vi "LS370Monitor.vi"() -> ()   [LabVIEW 2015]
uses:
  Instrument_Setup.vi
  Global/Global Variables/global.vi
  Global/Global Variables/Data_Display_global.vi
panel:
  out "Tsweeps Running":bool
  in  "Stopp":bool
  out "MC Heater Output":dbl
  # "Manuelle Steuerung"
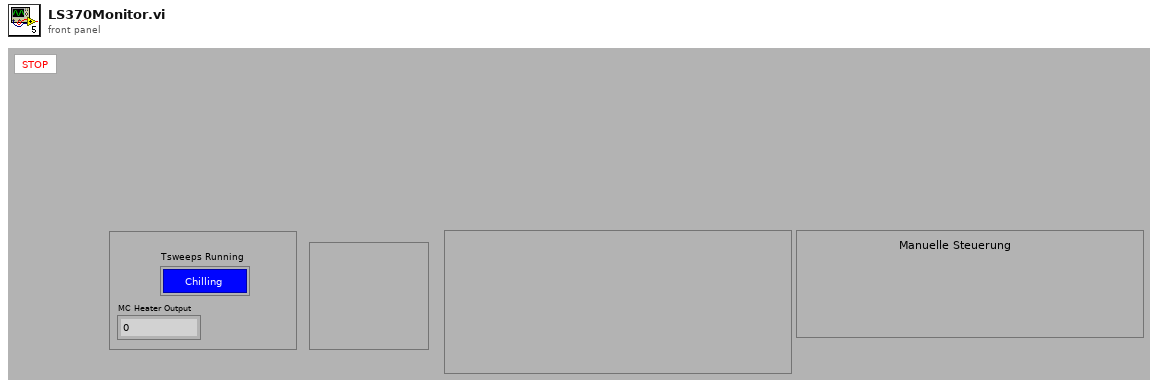
[diagram p1: front panel]
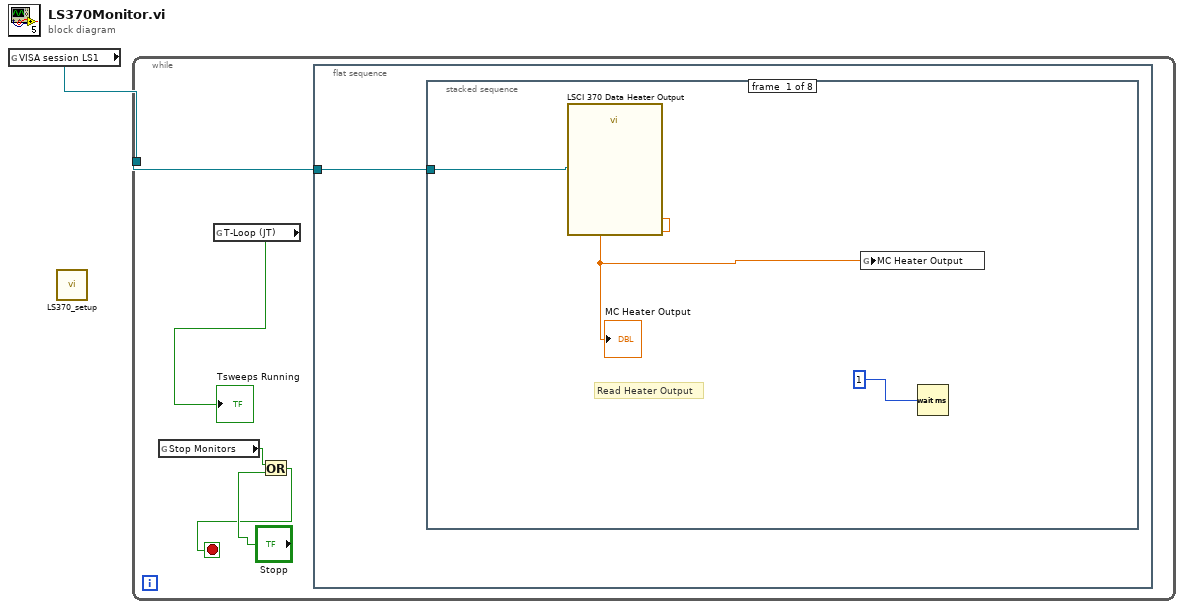
[diagram p0: block diagram]
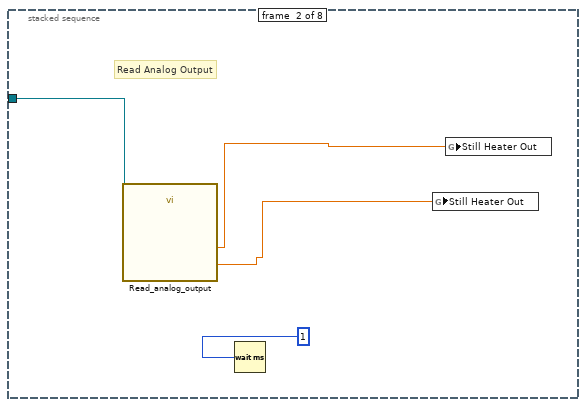
[diagram p2: hidden frame]
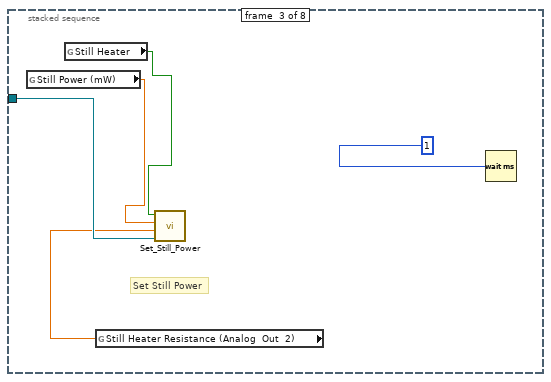
[diagram p3: hidden frame]
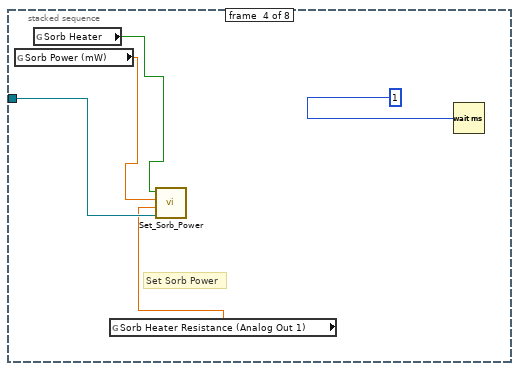
[diagram p4: hidden frame]
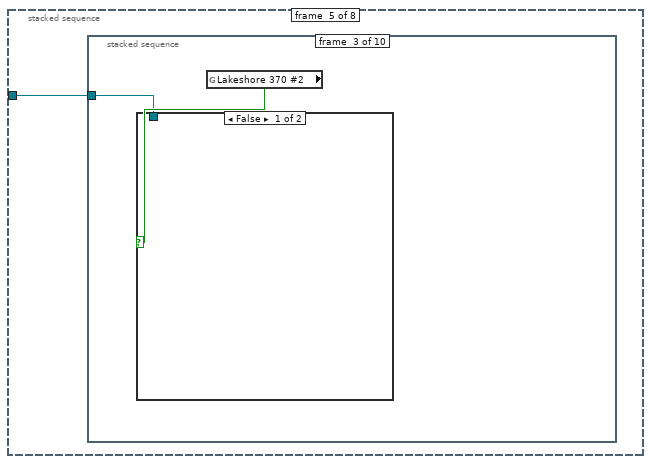
[diagram p5: hidden frame]
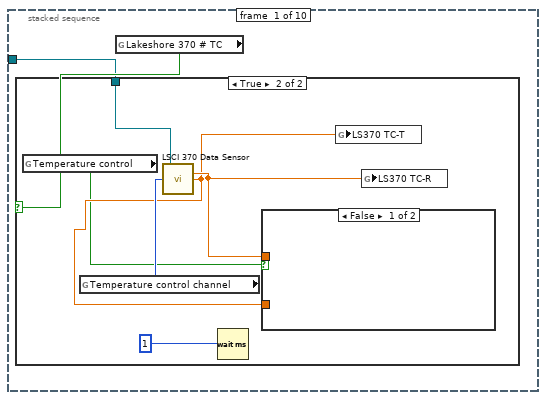
[diagram p6: hidden frame]
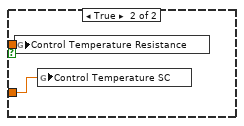
[diagram p8: hidden frame]
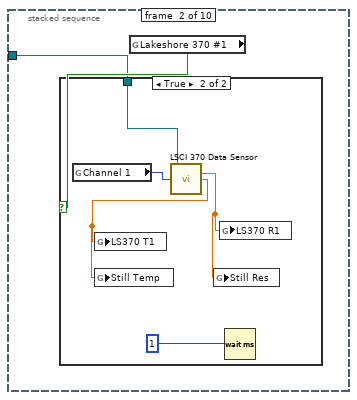
[diagram p9: hidden frame]
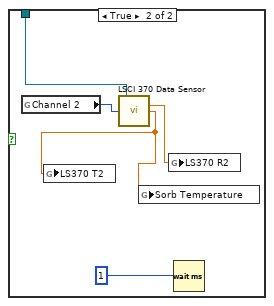
[diagram p11: hidden frame]
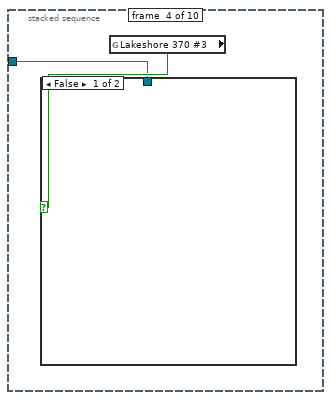
[diagram p12: hidden frame]
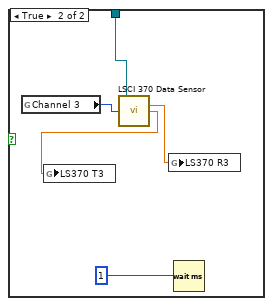
[diagram p13: hidden frame]
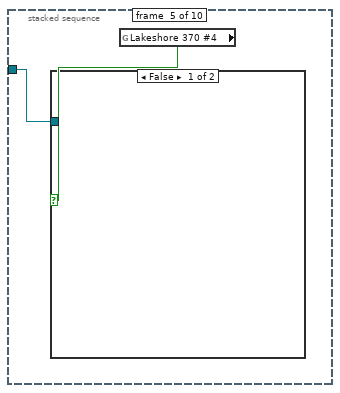
[diagram p14: hidden frame]
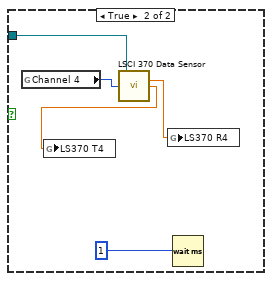
[diagram p15: hidden frame]
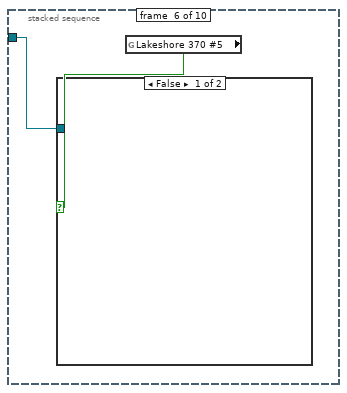
[diagram p16: hidden frame]
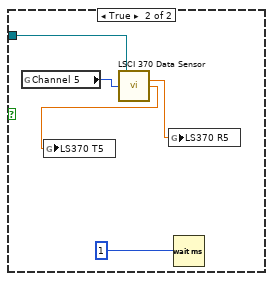
[diagram p17: hidden frame]
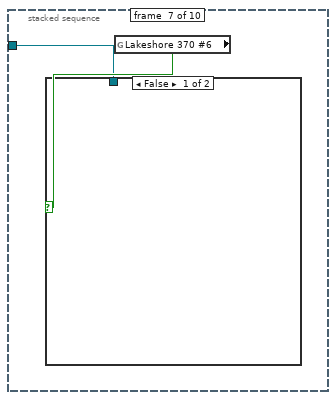
[diagram p18: hidden frame]
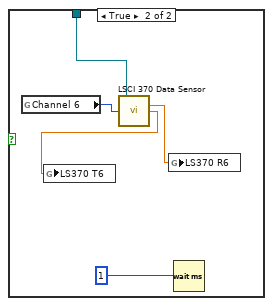
[diagram p19: hidden frame]
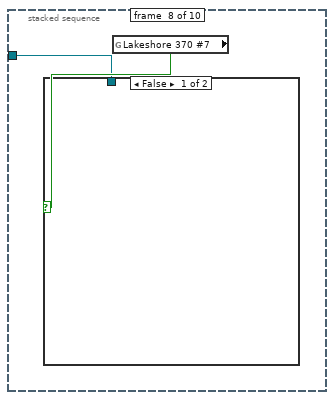
[diagram p20: hidden frame]
diagram:
  n1 = global read "Instrument_Setup.vi" "VISA session LS1"() -> (w1:refnum<visa-resource-name>)
  n2 = call "LS370_setup.vi"() -> ()  [unwired: 1 in]
  n3 = while {
    tunnel: w1 -> [w6]
    stop <- w2 stop-if-true
    n4 = global read "Data_Display_global.vi" "Stop Monitors"() -> (w4:bool)
    n5 = global read "global.vi" "T-Loop (JT)"() -> (→"Tsweeps Running":bool)
    n6 = Or(x=w4, y="Stopp") -> (x .or. y?=w2:bool)
    n7 = flat-sequence {
      tunnel: w6 -> [w7]
      frame #0 {
        n8 = stacked-sequence {
          tunnel: w7 -> [w10 w14 w19 w24 w25 _ _ _]
          frame #0 {
            # "Read Heater Output"
            n9 = call "LSCI 370 Data Heater Output.vi"("VISA session"=w10) -> ("Heater Output"=w9:dbl)  [unwired: 12 in, 2 out]
            "MC Heater Output" <- w9
            n10 = global write "Data_Display_global.vi" "MC Heater Output"(w9) -> ()
            n11 = Wait (ms)(milliseconds to wait=1) -> ()  [unwired: 1 out]
          }
          frame #1 {
            # "Read Analog Output"
            n12 = call "Read_analog_output.vi"("VISA session"=w14) -> ("Still Output"=w11:dbl, "Analog Output"=w12:dbl)  [unwired: 9 in]
            n13 = Wait (ms)(milliseconds to wait=1) -> ()  [unwired: 1 out]
            n14 = global write "Data_Display_global.vi" "Still Heater Out"(w11) -> ()
            n15 = global write "Data_Display_global.vi" "Still Heater Out"(w12) -> ()
          }
          frame #2 {
            # "Set Still Power"
            n16 = global read "Data_Display_global.vi" "Still Power (mW)"() -> (w15:dbl)
            n17 = global read "Data_Display_global.vi" "Still Heater"() -> (w16:bool)
            n18 = global read "Instrument_Setup.vi" "Still Heater Resistance (Analog  Out  2)"() -> (w18:dbl)
            n19 = call "Set_Still_Power.vi"("VISA session"=w19, "Still Heater Resistance (mW)"=w18, "Still Power (mW)"=w15, "Still heater"=w16) -> ()  [unwired: 8 in]
            n20 = Wait (ms)(milliseconds to wait=1) -> ()  [unwired: 1 out]
          }
          frame #3 {
            # "Set Sorb Power"
            n21 = global read "Data_Display_global.vi" "Sorb Power (mW)"() -> (w20:dbl)
            n22 = global read "Data_Display_global.vi" "Sorb Heater"() -> (w21:bool)
            n23 = global read "Instrument_Setup.vi" "Sorb Heater Resistance (Analog Out 1)"() -> (w23:dbl)
            n24 = call "Set_Sorb_Power.vi"("VISA session"=w24, "Sorb Heater Resistance (Ohm)"=w23, "Sorb Power (mW)"=w20, "Sorb heater"=w21) -> ()  [unwired: 8 in]
            n25 = Wait (ms)(milliseconds to wait=1) -> ()  [unwired: 1 out]
          }
          frame #4 {
            n26 = stacked-sequence {
              tunnel: w25 -> [w26 w36 w43 w50 w57 w64 w71 w78 w85 w92]
              frame #0 {
                n27 = global read "Instrument_Setup.vi" "Lakeshore 370 # TC"() -> (w27:bool)
                n28 = case shown="True" w27 {
                  tunnel: w26 -> [_ w31]
                  frame False {
                  }
                  frame True {
                    n29 = global read "Instrument_Setup.vi" "Temperature control"() -> (w28:bool)
                    n30 = global read "Instrument_Setup.vi" "Temperature control channel"() -> (w33:i32)
                    n31 = call "LSCI 370 Data Sensor.vi"("VISA session"=w31, "Channel (1)"=w33) -> ("Resistance Reading"=w30:dbl, "Kelvin Reading"=w29:dbl)  [unwired: 9 in, 3 out]
                    n32 = Wait (ms)(milliseconds to wait=1) -> ()  [unwired: 1 out]
                    n33 = case shown="False" w28 {
                      tunnel: w30 -> [_ w35]
                      tunnel: w29 -> [_ w34]
                      frame False {
                      }
                      frame True {
                        n34 = global write "Data_Display_global.vi" "Control Temperature Resistance"(w35) -> ()
                        n35 = global write "Data_Display_global.vi" "Control Temperature SC"(w34) -> ()
                      }
                    }
                    n36 = global write "Data_Display_global.vi" "LS370 TC-T"(w29) -> ()
                    n37 = global write "Data_Display_global.vi" "LS370 TC-R"(w30) -> ()
                  }
                }
              }
              frame #1 {
                n38 = global read "Instrument_Setup.vi" "Lakeshore 370 #1"() -> (w37:bool)
                n39 = case shown="True" w37 {
                  tunnel: w36 -> [_ w40]
                  frame False {
                  }
                  frame True {
                    n40 = global read "Instrument_Setup.vi" "Channel 1"() -> (w42:i32)
                    n41 = call "LSCI 370 Data Sensor.vi"("VISA session"=w40, "Channel (1)"=w42) -> ("Resistance Reading"=w39:dbl, "Kelvin Reading"=w38:dbl)  [unwired: 9 in, 3 out]
                    n42 = global write "Data_Display_global.vi" "LS370 T1"(w38) -> ()
                    n43 = global write "Data_Display_global.vi" "Still Temp"(w38) -> ()
                    n44 = global write "Data_Display_global.vi" "Still Res"(w39) -> ()
                    n45 = global write "Data_Display_global.vi" "LS370 R1"(w39) -> ()
                    n46 = Wait (ms)(milliseconds to wait=1) -> ()  [unwired: 1 out]
                  }
                }
              }
              frame #2 {
                n47 = global read "Instrument_Setup.vi" "Lakeshore 370 #2"() -> (w44:bool)
                n48 = case shown="False" w44 {
                  tunnel: w43 -> [_ w46]
                  frame False {
                  }
                  frame True {
                    n49 = global read "Instrument_Setup.vi" "Channel 2"() -> (w49:i32)
                    n50 = call "LSCI 370 Data Sensor.vi"("VISA session"=w46, "Channel (1)"=w49) -> ("Resistance Reading"=w47:dbl, "Kelvin Reading"=w45:dbl)  [unwired: 9 in, 3 out]
                    n51 = global write "Data_Display_global.vi" "LS370 T2"(w45) -> ()
                    n52 = global write "Data_Display_global.vi" "Sorb Temperature"(w45) -> ()
                    n53 = global write "Data_Display_global.vi" "LS370 R2"(w47) -> ()
                    n54 = Wait (ms)(milliseconds to wait=1) -> ()  [unwired: 1 out]
                  }
                }
              }
              frame #3 {
                n55 = global read "Instrument_Setup.vi" "Lakeshore 370 #3"() -> (w51:bool)
                n56 = case shown="False" w51 {
                  tunnel: w50 -> [_ w52]
                  frame False {
                  }
                  frame True {
                    n57 = global read "Instrument_Setup.vi" "Channel 3"() -> (w56:i32)
                    n58 = call "LSCI 370 Data Sensor.vi"("VISA session"=w52, "Channel (1)"=w56) -> ("Resistance Reading"=w53:dbl, "Kelvin Reading"=w54:dbl)  [unwired: 9 in, 3 out]
                    n59 = global write "Data_Display_global.vi" "LS370 T3"(w54) -> ()
                    n60 = global write "Data_Display_global.vi" "LS370 R3"(w53) -> ()
                    n61 = Wait (ms)(milliseconds to wait=1) -> ()  [unwired: 1 out]
                  }
                }
              }
              frame #4 {
                n62 = global read "Instrument_Setup.vi" "Lakeshore 370 #4"() -> (w58:bool)
                n63 = case shown="False" w58 {
                  tunnel: w57 -> [_ w59]
                  frame False {
                  }
                  frame True {
                    n64 = global read "Instrument_Setup.vi" "Channel 4"() -> (w63:i32)
                    n65 = call "LSCI 370 Data Sensor.vi"("VISA session"=w59, "Channel (1)"=w63) -> ("Resistance Reading"=w60:dbl, "Kelvin Reading"=w61:dbl)  [unwired: 9 in, 3 out]
                    n66 = global write "Data_Display_global.vi" "LS370 T4"(w61) -> ()
                    n67 = global write "Data_Display_global.vi" "LS370 R4"(w60) -> ()
                    n68 = Wait (ms)(milliseconds to wait=1) -> ()  [unwired: 1 out]
                  }
                }
              }
              frame #5 {
                n69 = global read "Instrument_Setup.vi" "Lakeshore 370 #5"() -> (w65:bool)
                n70 = case shown="False" w65 {
                  tunnel: w64 -> [_ w66]
                  frame False {
                  }
                  frame True {
                    n71 = global read "Instrument_Setup.vi" "Channel 5"() -> (w70:i32)
                    n72 = call "LSCI 370 Data Sensor.vi"("VISA session"=w66, "Channel (1)"=w70) -> ("Resistance Reading"=w67:dbl, "Kelvin Reading"=w68:dbl)  [unwired: 9 in, 3 out]
                    n73 = global write "Data_Display_global.vi" "LS370 T5"(w68) -> ()
                    n74 = global write "Data_Display_global.vi" "LS370 R5"(w67) -> ()
                    n75 = Wait (ms)(milliseconds to wait=1) -> ()  [unwired: 1 out]
                  }
                }
              }
              frame #6 {
                n76 = global read "Instrument_Setup.vi" "Lakeshore 370 #6"() -> (w72:bool)
                n77 = case shown="False" w72 {
                  tunnel: w71 -> [_ w73]
                  frame False {
                  }
                  frame True {
                    n78 = global read "Instrument_Setup.vi" "Channel 6"() -> (w77:i32)
                    n79 = call "LSCI 370 Data Sensor.vi"("VISA session"=w73, "Channel (1)"=w77) -> ("Resistance Reading"=w74:dbl, "Kelvin Reading"=w75:dbl)  [unwired: 9 in, 3 out]
                    n80 = global write "Data_Display_global.vi" "LS370 T6"(w75) -> ()
                    n81 = global write "Data_Display_global.vi" "LS370 R6"(w74) -> ()
                    n82 = Wait (ms)(milliseconds to wait=1) -> ()  [unwired: 1 out]
                  }
                }
              }
              frame #7 {
                n83 = global read "Instrument_Setup.vi" "Lakeshore 370 #7"() -> (w79:bool)
                n84 = case shown="False" w79 {
                  tunnel: w78 -> [_ w80]
                  frame False {
                  }
                  frame True {
                    n85 = global read "Instrument_Setup.vi" "Channel 7"() -> (w84:i32)
                    n86 = call "LSCI 370 Data Sensor.vi"("VISA session"=w80, "Channel (1)"=w84) -> ("Resistance Reading"=w81:dbl, "Kelvin Reading"=w82:dbl)  [unwired: 9 in, 3 out]
                    n87 = global write "Data_Display_global.vi" "LS370 T7"(w82) -> ()
                    n88 = global write "Data_Display_global.vi" "LS370 R7"(w81) -> ()
                    n89 = Wait (ms)(milliseconds to wait=1) -> ()  [unwired: 1 out]
                  }
                }
              }
              frame #8 {
                n90 = global read "Instrument_Setup.vi" "Lakeshore 370 #8"() -> (w86:bool)
                n91 = case shown="False" w86 {
                  tunnel: w85 -> [_ w87]
                  frame False {
                  }
                  frame True {
                    n92 = global read "Instrument_Setup.vi" "Channel 8"() -> (w91:i32)
                    n93 = call "LSCI 370 Data Sensor.vi"("VISA session"=w87, "Channel (1)"=w91) -> ("Resistance Reading"=w88:dbl, "Kelvin Reading"=w89:dbl)  [unwired: 9 in, 3 out]
                    n94 = global write "Data_Display_global.vi" "LS370 T8"(w89) -> ()
                    n95 = global write "Data_Display_global.vi" "LS370 R8"(w88) -> ()
                    n96 = Wait (ms)(milliseconds to wait=1) -> ()  [unwired: 1 out]
                  }
                }
              }
              frame #9 {
                n97 = global read "Instrument_Setup.vi" "Lakeshore 370 #9"() -> (w93:bool)
                n98 = case shown="False" w93 {
                  tunnel: w92 -> [_ w94]
                  frame False {
                  }
                  frame True {
                    n99 = global read "Instrument_Setup.vi" "Channel 9"() -> (w98:i32)
                    n100 = call "LSCI 370 Data Sensor.vi"("VISA session"=w94, "Channel (1)"=w98) -> ("Resistance Reading"=w95:dbl, "Kelvin Reading"=w96:dbl)  [unwired: 9 in, 3 out]
                    n101 = global write "Data_Display_global.vi" "LS370 T9"(w96) -> ()
                    n102 = global write "Data_Display_global.vi" "LS370 R9"(w95) -> ()
                    n103 = Wait (ms)(milliseconds to wait=1) -> ()  [unwired: 1 out]
                  }
                }
              }
            }
          }
          frame #5 {
            n104 = global read "Data_Display_global.vi" "Update LS"() -> (w99:bool)
            n105 = case shown="False" w99 {
              frame False {
              }
              frame True {
                n106 = flat-sequence {
                  frame #0 {
                    n107 = call "LS370_setup.vi"() -> ()  [unwired: 1 in]
                    n108 = Wait (ms)(milliseconds to wait=1) -> ()  [unwired: 1 out]
                  }
                }
              }
            }
          }
          frame #6 {
            n109 = flat-sequence {
              frame #0 {
                n110 = global read "global.vi" "Set JT Temperature Sweep"() -> (w102:bool)
                n111 = case shown="False" w102 {
                  tunnel: [w106 w115] -> w101
                  frame False {
                    n112 = global read "Data_Display_global.vi" "Setpoint - Manual"() -> (w104:dbl)
                    n113 = global read "Data_Display_global.vi" "Activate Tsweep"() -> (w105:bool)
                    n114 = global read "Data_Display_global.vi" "Rate (K/min)"() -> (w103:dbl)
                    n115 = case shown="False" w105 {
                      tunnel: w104 -> [_ w113]
                      tunnel: w103 -> [_ w114]
                      tunnel: [w107 w113] -> w106
                      frame False {
                        n116 = global read "global.vi" "Cerrent State"() -> (w110:i32)
                        n117 = Equal?(x=1, y=w110) -> (x = y?=w108:bool)
                        n118 = case shown="False" w108 {
                          tunnel: [w111 w112] -> w107
                          frame False {
                            n119 = global read "global.vi" "T final (K)"() -> (w111:dbl)
                          }
                          frame True {
                            n120 = global read "global.vi" "T init. (K)"() -> (w112:dbl)
                          }
                        }
                      }
                      frame True {
                        n121 = call "Start_Sweep_Manual.vi"("Rate"=w114, "Setpoint"=w113) -> ()  [unwired: 10 in]
                      }
                    }
                  }
                  frame True {
                    n122 = call "Start_Ramping.vi"() -> ("Setpoint"=w115:dbl)  [unwired: 11 in]
                    n123 = Wait (ms)(milliseconds to wait=1) -> ()  [unwired: 1 out]
                  }
                }
                n124 = global write "Data_Display_global.vi" "Setpoint"(w101) -> ()
              }
              frame #1 {
                w117 = FALSE
                n125 = global write "global.vi" "Set JT Temperature Sweep"(w117) -> ()
                n126 = global write "Data_Display_global.vi" "Activate Tsweep"(w117) -> ()
              }
            }
          }
          frame #7 {
            n127 = flat-sequence {
              frame #0 {
                n128 = global read "Data_Display_global.vi" "Disable Heater"() -> (w118:bool)
                n129 = case shown="True" w118 {
                  frame False {
                  }
                  frame True {
                    n130 = flat-sequence {
                      frame #0 {
                        n131 = call "Disable_Zone_Tuning.vi"() -> ()  [unwired: 1 in]
                        n132 = Wait (ms)(milliseconds to wait=10) -> ()  [unwired: 1 out]
                      }
                      frame #1 {
                        n133 = global write "Data_Display_global.vi" "Disable Heater"(FALSE) -> ()
                      }
                    }
                  }
                }
              }
              frame #1 {
                n134 = global write "global.vi" "Disable Zone Tuning"(FALSE) -> ()
              }
            }
          }
        }
      }
    }
  }
